vi "RT Start.vi"(8 "error in (no error)":errorcluster, 11 "1553 Unit Test in":refnum<class "Remote Terminal.lvclass">) -> (0 "error out":errorcluster, 3 "1553 Unit Test out":refnum<class "Remote Terminal.lvclass">)   [LabVIEW 2020, in "Unit Tests.lvlib" / "Remote Terminal.lvclass"]
uses:
  Remote Terminal.lvclass
  Remote Terminal.lvclass/Remote Terminal.ctl
  <vilib>/addons/_JKI Toolkits/Caraya/classes/Assert/Assert True.vi
  1553 Session/1553 Session.lvclass
  Dependencies/FPGA Interface/FPGA Interface.lvclass
  <vilib>/addons/_JKI Toolkits/Caraya/classes/Test/Test.lvclass
  <vilib>/addons/_JKI Toolkits/Caraya/classes/Assert/Assert.lvclass
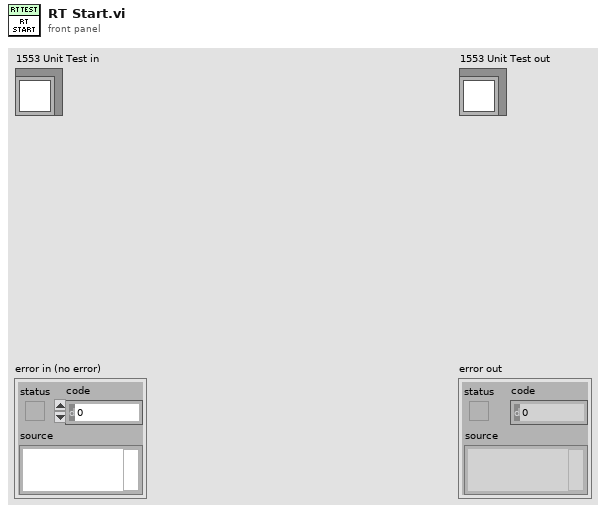
[diagram p1: front panel]
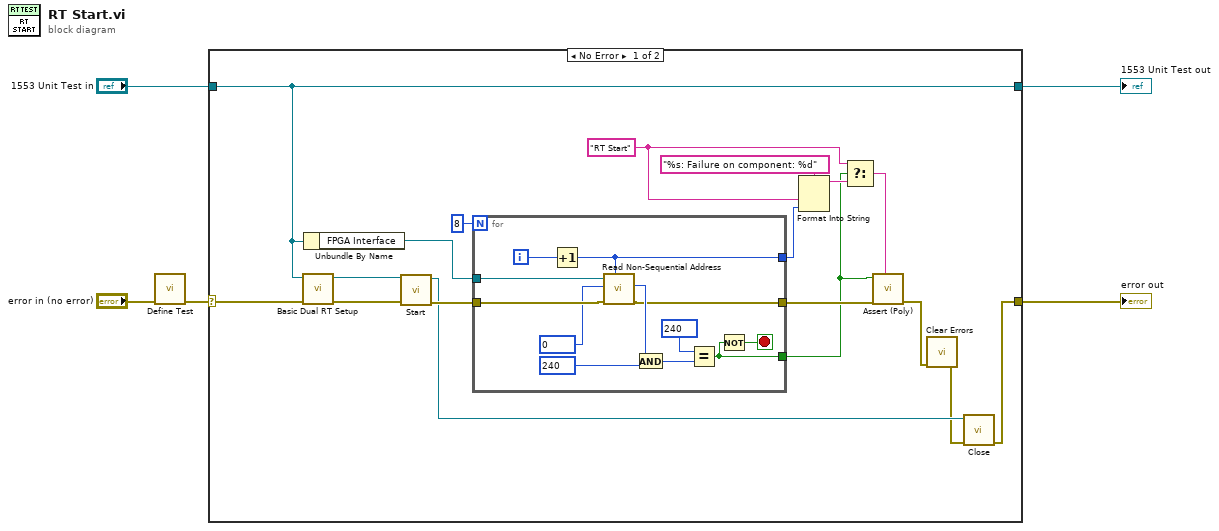
[diagram p0: block diagram]
diagram:
  n1 = call <vilib>:"Define Test.vi"("error in (no error)"="error in (no error)") -> ("error out"=w2:errorcluster)  [unwired: 9 in, 1 out]
  n2 = case shown="No Error" w2 {
    selector: w2 -> [w20 w37]
    tunnel: [w6 w37] -> w5
    tunnel: [w10 w36] -> w3
    tunnel: "1553 Unit Test in" -> [w10 w36]
    frame No Error {
      w12 = "RT Start" ("custom report message (\"\")")
      n3 = call "Basic Dual RT Setup.vi"("error in (no error)"=w20, "1553 Unit Test in"=w10) -> ("error out"=w19:errorcluster, "1553 Session out"=w9:refnum<class "1553 Session.lvclass">)  [unwired: 8 in]
      n4 = Unbundle By Name(w10) -> ("FPGA Interface"=w16:refnum<class "FPGA Interface.lvclass">)
      n5 = call-dynamic "Start.vi"("error in (no error)"=w19, "1553 Board in"=w9) -> ("error out"=w17:errorcluster, "1553 Board out"=w11:refnum<class "1553 Session.lvclass">)  [unwired: 8 in]
      n6 = for {
        N: 8 -> [_]
        tunnel: w16 -> [w31]
        tunnel: w17 -> [w30]
        tunnel: [w25] -> w14
        tunnel: [w29] -> w13
        tunnel: [w26] -> w15
        i -> [w35]
        stop <- w24 stop-if-true
        n7 = Increment(x=w35) -> (x+1=w29:i32)
        n8 = call-dynamic "Read Non-Sequential Address.vi"("Target IC (1-8)"=w29, "error in (no error)"=w30, "Address"=u16 0, "FPGA Interface in"=w31) -> ("error out"=w26:errorcluster, "Data"=w27:u16)  [unwired: 6 in]
        n9 = And(x=w27, y=u16 240) -> (x .and. y?=w32:u16)
        n10 = Equal?(x=u16 240, y=w32) -> (x = y?=w25:bool)
        n11 = Not(x=w25) -> (.not. x?=w24:bool)
      }
      n12 = Format Into String(format string="%s: Failure on component: %d" ("custom report message (\"\")"), w12, w13) -> (resulting string=w22:string)  [unwired: 2 in, 1 out]
      n13 = Select(t=w12, s=w14, f=w22) -> (s? t:f=w21:string)
      n14 = call-poly <vilib>:"Assert (Poly).vi"("Label"=w21, "error in (no error)"=w15, "True?"=w14) -> ("error out"=w8:errorcluster)  [unwired: 7 in, 1 out]
      n15 = call <vilib>:"Clear Errors.vi"("error in (no error)"=w8) -> ("error out"=w7:errorcluster)  [unwired: 5 in, 1 out]
      n16 = call-dynamic "Close.vi"("error in (no error)"=w7, "1553 Board in"=w11) -> ("error out"=w6:errorcluster)  [unwired: 9 in]
    }
    frame Error {
    }
  }
  "error out" <- w5
  "1553 Unit Test out" <- w3
